vi "Connect SDK.vi"() -> ()   [LabVIEW 2025]
uses:
  ExtremelyEpicImagerIPC2.lvlib
panel:
  in  "Set Fixed Emissivity":sgl
  out "Fixed Emissivity":sgl
  in  "stop":bool
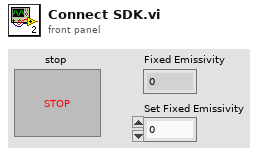
[diagram p1: front panel]
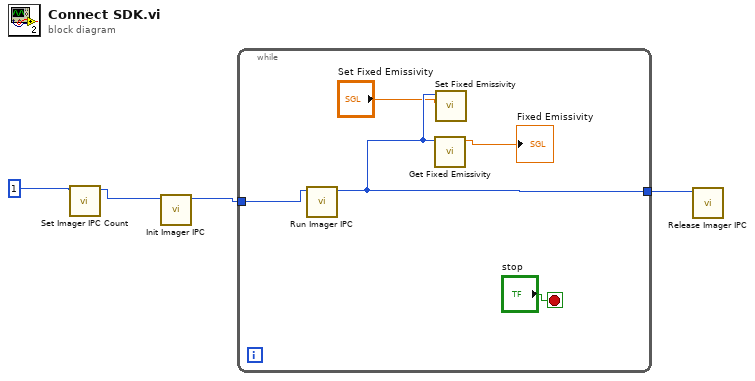
[diagram p0: block diagram]
diagram:
  n1 = call "Set Imager IPC Count.vi"("count"=u16 1) -> ("function return"=w4:i32)  [unwired: 10 in]
  n2 = call "Init Imager IPC.vi"("index"=w4) -> ("function return"=w2:i32)  [unwired: 10 in]
  n3 = while {
    tunnel: w2 -> [w9]
    tunnel: [w6] -> w1
    stop <- "stop" stop-if-true
    n4 = call "Run Imager IPC.vi"("index"=w9) -> ("function return"=w6:i32)  [unwired: 10 in]
    n5 = call "Get Fixed Emissivity.vi"("index"=w6) -> ("function return"=→"Fixed Emissivity":sgl)  [unwired: 10 in]
    n6 = call "Set Fixed Emissivity.vi"("Value"="Set Fixed Emissivity", "index"=w6) -> ()  [unwired: 9 in, 1 out]
  }
  n7 = call "Release Imager IPC.vi"("index"=w1) -> ()  [unwired: 10 in, 1 out]
